vi "FROG_GenerateTemplate.vi"(3 "Delay Info":T1={"Delay Temporal Resolution"=120, "Delay Spatial Resolution"=300}, 4 "Spectrum Info":T2={"Wavelength Max"=552.65689, "Wavelength Min"=252.4975, "Spectrum Resolution"=1143}) -> (0 "Time Scale":cluster{"Time Multplier":dbl, "Time Offset":dbl}, 1 "Time Array":dbl[](array[numeric]), 2 "Noise Array":dbl[](array[numeric]))   [LabVIEW 2013]
uses:
  <vilib>/Analysis/NI_AALBase.lvlib
panel:
  in  "Numeric Rnd?":bool
  out "Time Multiplier":dbl
  out "Time Offset":dbl
  in  "Seed":u16
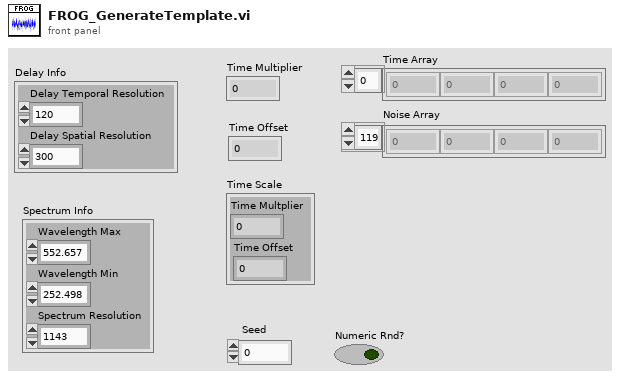
[diagram p1: front panel]
types:
  T1 = cluster{"Delay Temporal Resolution":u16, "Delay Spatial Resolution":u16}
  T2 = cluster{"Wavelength Max":dbl, "Wavelength Min":dbl, "Spectrum Resolution":u16}
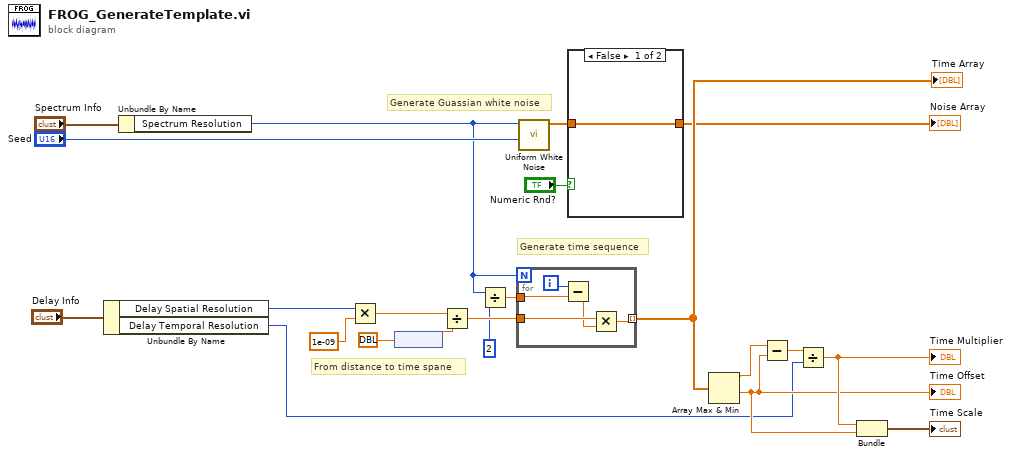
[diagram p0: block diagram]
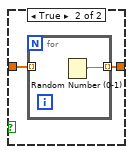
[diagram p2: hidden frame]
diagram:
  # "Generate Guassian white noise"
  # "Generate time sequence"
  # "From distance to time spane"
  n1 = Unbundle By Name("Delay Info") -> ("Delay Spatial Resolution"=w6:u16, "Delay Temporal Resolution"=w4:u16)
  n2 = Unbundle By Name("Spectrum Info") -> ("Spectrum Resolution"=w8:u16)
  n3 = Multiply(x=w6, y=1e-09) -> (x*y=w20:dbl)
  n4 = node(ext[unit] 299792458.0) -> (w18:ext)
  n5 = Divide(x=w20, y=w18) -> (x/y=w21:ext)
  n6 = Divide(x=w8, y=2) -> (x/y=w15:dbl)
  n7 = for {
    N: w8 -> [_]
    tunnel: [w26] -> w5 mode=indexing
    tunnel: w21 -> [w27]
    tunnel: w15 -> [w23]
    i -> [w25]
    n8 = Subtract(x=w25, y=w23) -> (x-y=w24:dbl)
    n9 = Multiply(x=w27, y=w24) -> (x*y=w26:ext)
  }
  "Time Array" <- w5
  n10 = call <vilib>:"Uniform White Noise.vi"("seed"="Seed", "samples"=w8) -> ("uniform white noise"=w3:dbl[])  [unwired: 8 in, 1 out]
  n11 = case shown="False" "Numeric Rnd?" {
    tunnel: w3 -> [w28 w30]
    tunnel: [w28 w29] -> w2
    frame False {
    }
    frame True {
      n12 = for {
        tunnel: w30 -> [_] mode=indexing
        tunnel: [w31] -> w29 mode=indexing
        n13 = Random Number (0-1)() -> (number: 0 to 1=w31:dbl)
      }
    }
  }
  "Noise Array" <- w2
  n14 = Array Max & Min(array=w5) -> (max value=w10:ext, min value=w11:ext)  [unwired: 2 out]
  "Time Offset" <- w11
  n15 = Subtract(x=w10, y=w11) -> (x-y=w13:ext)
  n16 = Divide(x=w13, y=w4) -> (x/y=w12:ext)
  "Time Multiplier" <- w12
  n17 = Bundle(w12, w11) -> (→"Time Scale":cluster{ext, ext})  [unwired: 1 in]
